vi "BMU参数读取-Auto.vi"(7 "Socket":dbl, 8 "CAN端口":u16(ring), 9 "设备索引号":u16(ring), 10 "CAN卡类型":u32(ring)=21, 11 "从板号":u8=1) -> (3 "成功?":bool)   [LabVIEW 2013] (continued)
                                tunnel: w3912 -> [w3927] mode=indexing
                                tunnel: [w3923] -> w3910 mode=indexing
                                n2326 = Equal To 0?(x=w3927) -> (x = 0?=w3926:bool)
                                n2327 = Select(t="无", s=w3926, f="故障") -> (s? t:f=w3923:string)
                                }
                                n2328 = Insert Into Array(array=w3911, new element=w3910) -> (w3909:string[])  [unwired: 1 in]
                              }
                              n2329 = call "详细故障分解.vi"("名称"=string[] ["初始化失败(RS232)", "发送异常(RS232)", "接收异常(RS232)", "总线超时(RS232)", "初始化失败(RS485)", "发送异常(RS485)", "接收异常(RS485)", "总线超时(RS485)"], "故障输入口"=w3903) -> ("输出数组"=w3901:string[][])  [unwired: 1 in, 2 out]
                              n2330 = local write "电池故障"(w3901) -> ()
                            }
                            frame 6 {
                              n2331 = for {
                                N: 2 -> [_]
                                tunnel: w3932 -> [w3949]
                                shift-right: [w3936] -> w3930
                                shift-left: string[] [] -> [w3938]
                                i -> [w3935]
                                w3943 = 8 ("索引")
                                w3947 = 2 ("y")
                                n2332 = Multiply(x=w3935, y=w3947) -> (x*y=w3948:i32)
                                n2333 = Array Subset(array=w3949, index=w3948, length=w3947) -> (w3946:u8[])
                                n2334 = Index Array(array=w3946) -> (element #1=w3945:u8, element #2=w3944:u8)  [unwired: 2 in]
                                n2335 = call "二进制解析-8.6.vi"("索引"=w3943, "数值"=w3945) -> ("低位子数组"=w3942:i32[])  [unwired: 1 in, 2 out]
                                n2336 = call "二进制解析-8.6.vi"("索引"=w3943, "数值"=w3944) -> ("低位子数组"=w3941:i32[])  [unwired: 1 in, 2 out]
                                n2337 = Insert Into Array(array=w3942, new element=w3941) -> (w3940:i32[])  [unwired: 1 in]
                                n2338 = Reverse 1D Array(array=w3940) -> (reversed array=w3939:i32[])
                                n2339 = for {
                                N: 16 -> [_]
                                tunnel: w3939 -> [w3954] mode=indexing
                                tunnel: [w3950] -> w3937 mode=indexing
                                n2340 = Equal To 0?(x=w3954) -> (x = 0?=w3953:bool)
                                n2341 = Select(t="无", s=w3953, f="故障") -> (s? t:f=w3950:string)
                                }
                                n2342 = Insert Into Array(array=w3938, new element=w3937) -> (w3936:string[])  [unwired: 1 in]
                              }
                              n2343 = call "详细故障分解.vi"("名称"=string[] ["DI1对地短", "DI1对电源短", "DI2对地短", "DI2对电源短", "DI3对地短", "DI3对电源短", "DI4对地短", "DI4对电源短", "DI5对地短", "DI5对电源短", "DI6对地短", "DI6对电源短", "DI7对地短", "DI7对电源短", "DI8对地短", "DI8对电源短", "DO1对地短", "DO1对电源短", "DO2对地短", "DO2对电源短", "DO3对地短", "DO3对电源短", "DO4对地短", "DO4对电源短", "DO5对地短", "DO5对电源短", "DO6对地短", "DO6对电源短", "DO7对地短", "DO7对电源短", "DO8对地短", "DO8对电源短"], "故障输入口"=w3930) -> ("输出数组"=w3928:string[][])  [unwired: 1 in, 2 out]
                              n2344 = local write "电池故障"(w3928) -> ()
                            }
                            frame 7 {
                              n2345 = for {
                                N: 2 -> [_]
                                tunnel: w3959 -> [w3976]
                                shift-right: [w3963] -> w3957
                                shift-left: string[] [] -> [w3965]
                                i -> [w3961]
                                w3970 = 8 ("索引")
                                w3974 = 2 ("y")
                                n2346 = Multiply(x=w3961, y=w3974) -> (x*y=w3975:i32)
                                n2347 = Array Subset(array=w3976, index=w3975, length=w3974) -> (w3973:u8[])
                                n2348 = Index Array(array=w3973) -> (element #1=w3972:u8, element #2=w3971:u8)  [unwired: 2 in]
                                n2349 = call "二进制解析-8.6.vi"("索引"=w3970, "数值"=w3972) -> ("低位子数组"=w3969:i32[])  [unwired: 1 in, 2 out]
                                n2350 = call "二进制解析-8.6.vi"("索引"=w3970, "数值"=w3971) -> ("低位子数组"=w3968:i32[])  [unwired: 1 in, 2 out]
                                n2351 = Insert Into Array(array=w3969, new element=w3968) -> (w3967:i32[])  [unwired: 1 in]
                                n2352 = case shown="1" w3961 {
                                tunnel: [4 6] -> w3962
                                frame 0, Default {
                                }
                                frame 1 {
                                }
                                }
                                n2353 = Reverse 1D Array(array=w3967) -> (reversed array=w3966:i32[])
                                n2354 = for {
                                N: w3962 -> [_]
                                tunnel: w3966 -> [w3983] mode=indexing
                                tunnel: [w3979] -> w3964 mode=indexing
                                n2355 = Equal To 0?(x=w3983) -> (x = 0?=w3982:bool)
                                n2356 = Select(t="无", s=w3982, f="故障") -> (s? t:f=w3979:string)
                                }
                                n2357 = Insert Into Array(array=w3965, new element=w3964) -> (w3963:string[])  [unwired: 1 in]
                              }
                              n2358 = call "详细故障分解.vi"("名称"=string[] ["超时(pre-chg)", "后端开路(pre-chg)", "后端短路(pre-chg)", "预充电回路断开(pre-chg)", "正级继电器驱动故障(relay_driver)", "负级继电器驱动故障(relay_driver)", "预充电继电器驱动故障(relay_driver)", "充电继电器驱动故障(relay_driver)", "风机继电器驱动故障(relay_driver)", "加热继电器驱动故障(relay_driver)"], "故障输入口"=w3957) -> ("输出数组"=w3955:string[][])  [unwired: 1 in, 2 out]
                              n2359 = local write "电池故障"(w3955) -> ()
                            }
                          }
                        }
                        frame True {
                          n2360 = Index Array(array=w3987, index #1=0 ("索引"), index #2=1 ("索引")) -> (element #1=w3990:u8, element #2=w3991:u8)
                          n2361 = Join Numbers(hi=w3990, lo=w3991) -> ((hi.lo)=w3989:u16)
                          n2362 = Number To Hexadecimal String(2:w3989) -> (0:w3988:string)  [unwired: 1 out]
                          n2363 = Concatenate Strings("读取错误，代码： " ("字符串"), "0x" ("字符串"), w3988) -> (w3986:string)
                          n2364 = One Button Dialog(message=w3986, button name ("OK")="是" ("按钮名称（“确定”）")) -> ()  [unwired: 1 out]
                        }
                      }
                      n2365 = local write "消除"(FALSE ("消除")) -> ()
                      n2366 = global write "EV05全局变量1.vi" "流控帧 2"(FALSE ("流控帧 2")) -> ()
                      n2367 = local write "控制1"(FALSE ("控制1")) -> ()
                      n2368 = global write "EV05全局变量1.vi" "写入超时"(TRUE ("写入超时")) -> ()
                    }
                  }
                }
              }
            }
          }
        }
      }
      frame Error {
      }
    }
  }
  n2369 = disable-structure shown="启用" {
    disable-tunnel: w37 -> [w4002 _]
    disable-tunnel: w29 -> [w3997 _]
    disable-tunnel: w26 -> [w3996 _]
    disable-tunnel: w6 -> [w3995 _]
    frame Disabled {
      n2370 = while {
        tunnel: w4002 -> [w4011]
        tunnel: w3995 -> [w4010]
        tunnel: [w4009] -> w4001
        tunnel: [w4008] -> w4000
        tunnel: w3997 -> [_]
        tunnel: w3996 -> [_]
        stop <- w4007 stop-if-true
        n2371 = event shown="[49] \"全部读取\": 值改变" {
          selector: _ -> [_ _ _ _ _ _ _ _ _ _ _ _ _ _ _ _ _ _ _ _ _ _ _ _ _ _ _ _ _ _ _ _ _ _ _ _ _ _ _ _ _ _ _ _ _ _ _ _ _ _ _ _ _]
          dyn-events: _ -> [_ _ _ _ _ _ _ _ _ _ _ _ _ _ _ _ _ _ _ _ _ _ _ _ _ _ _ _ _ _ _ _ _ _ _ _ _ _ _ _ _ _ _ _ _ _ _ _ _ _ _ _ _]
          timeout: 200 -> [_ _ _ _ _ _ _ _ _ _ _ _ _ _ _ _ _ _ _ _ _ _ _ _ _ _ _ _ _ _ _ _ _ _ _ _ _ _ _ _ _ _ _ _ _ _ _ _ _ _ _ _ _]
          tunnel: [_ w4014 w4054 _ _ _ _ _ _ _ _ _ _ _ _ _ _ _ _ _ _ _ _ _ _ _ _ _ _ _ _ _ _ _ _ _ _ _ _ _ _ _ _ _ _ _ _ _ _ _ _ _ _] -> w4006
          tunnel: w4011 -> [w4013 w4017 w4053 _ w4094 w4105 w4116 w4127 w4132 w4143 w4154 w4165 w4176 w4187 w4204 w4215 w4231 w4769 w5191 w5216 w5244 w5347 w5420 w5432 w5442 w5488 _ _ w5538 w5605 w5672 w5739 w5806 w5873 w5940 w6008 w6076 w6143 w6210 w6280 w6291 w6330 w6352 w6392 w6414 w6452 w6512 w6547 w6583 w6616 w6685 w6718 w6751]
          tunnel: w4010 -> [w4012 w4016 w4052 _ w4093 w4104 w4115 w4126 w4131 w4142 w4153 w4164 w4175 w4186 w4203 w4214 w4230 w4768 w5190 w5215 w5243 w5346 w5418 w5430 w5441 w5487 _ _ w5537 w5604 w5671 w5738 w5805 w5872 w5939 w6007 w6075 w6142 w6209 w6278 w6290 w6329 w6351 w6391 w6413 w6451 w6511 w6546 w6582 w6615 w6684 w6717 w6750]
          tunnel: [w4013 w4017 w4053 _ w4094 w4105 w4116 w4127 w4132 w4143 w4154 w4165 w4176 w4187 w4204 w4215 w4231 w4769 w5191 w5216 w5244 w5347 w5419 w5431 w5442 w5488 _ _ w5538 w5605 w5672 w5739 w5806 w5873 w5940 w6008 w6076 w6143 w6210 w6279 w6289 w6328 w6350 w6390 w6412 w6452 w6510 w6545 w6581 w6614 w6683 w6716 w6749] -> w4009
          tunnel: [w4012 w4016 w4052 _ w4093 w4104 w4115 w4126 w4131 w4142 w4153 w4164 w4175 w4186 w4203 w4214 w4230 w4768 w5190 w5215 w5243 w5346 w5417 w5429 w5441 w5487 _ _ w5537 w5604 w5671 w5738 w5805 w5872 w5939 w6007 w6075 w6142 w6209 w6277 w6288 w6327 w6349 w6389 w6411 w6451 w6509 w6544 w6580 w6613 w6682 w6715 w6748] -> w4008
          tunnel: [_ _ _ _ _ _ _ _ _ _ _ _ _ _ _ _ _ _ _ _ _ _ _ _ _ _ _ _ _ _ _ _ _ _ _ _ _ _ _ _ w6288 w6327 w6349 w6389 w6411 _ w6509 w6544 w6580 w6613 w6682 w6715 w6748] -> w4005
          event Timeout {
            n2372 = event-data() -> ()  [unwired: 3 out]
          }
          event "停止": Value Change {
            n2373 = event-data() -> ("NewVal"=w4015:bool)  [unwired: 5 out]
            n2374 = stacked-sequence {
              tunnel: w4015 -> [w4034 _]
              tunnel: [w4034 _] -> w4014
              frame #0 {
                n2375 = global read "配置文件全局.vi" "诊断标定读取地址"() -> (w4018:path)
                n2376 = call <vilib>:"Application Directory.vi"() -> ("Application Directory"=w4028:path)
                n2377 = property class="VI"("FP.State"=T30."Hidden" ("前面板窗口:状态")) -> (reference out=w4030:refnum<vi>, error out=w4029:errorcluster)  [unwired: 2 in]
                n2378 = Build Path(base path=w4028, name or relative path="config.ini" ("名称或相对路径")) -> (appended path=w4026:path)
                n2379 = call <vilib>:"Open Config Data.vi"("configuration file path"=w4026) -> ("error out"=w4023:errorcluster, "refnum"=w4025:T26)  [unwired: 8 in, 1 out]
                n2380 = local write "停止"(TRUE ("停止")) -> ()
                n2381 = property class="VI"(reference=w4030, error in=w4029, "Front Panel.Open"=FALSE ("前面板窗口:打开")) -> ()  [unwired: 2 out]
                n2382 = call-poly <vilib>:"Write Key.vi"("section"="总信息", "error in (no error)"=w4023, "value"=w4018, "key"="诊断标定读取地址" ("section"), "refnum"=w4025) -> ("error out"=w4022:errorcluster, "refnum out"=w4021:T26)  [unwired: 4 in, 1 out]
                n2383 = call <vilib>:"Close Config Data.vi"("error in (no error)"=w4022, "refnum"=w4021) -> ("error out"=w4020:errorcluster)  [unwired: 8 in, 1 out]
                n2384 = call <vilib>:"Clear Errors.vi"("error in (no error)"=w4020) -> ()  [unwired: 6 in, 1 out]
              }
              frame #1 {
                n2385 = disable-structure shown="禁用" {
                  frame Disabled {
                    n2386 = local read "设备索引号"() -> (w4040:u16)
                    n2387 = local read "CAN卡类型"() -> (w4041:u32)
                    n2388 = local read "CAN端口"() -> (w4039:u16)
                    n2389 = Build Array(7) -> (w4036:i32[])
                    n2390 = call "transmit-8.6.vi"("can卡类型"=w4041, "设备索引号"=w4040, "CAN端口"=w4039, "ID"=418398080, "SendType"=u8 0, "Data"=w4036) -> ()  [unwired: 3 in, 11 out]
                  }
                  frame Enabled {
                    w4048 = u8 0 items=["Normal", "Listen Only"] ("工作方式")
                    w4047 = u8 1 items=["Dual Filter", "Single Filter"] ("滤波方式")
                    n2391 = local read "设备索引号"() -> (w4043:u16)
                    n2392 = local read "CAN卡类型"() -> (w4042:u32)
                    n2393 = local read "CAN端口"() -> (w4044:u16)
                    n2394 = call "CAN_Init-8.6.vi"("CAN卡类型"=w4042, "设备索引号"=w4043, "CAN端口"=w4044, "操作类型"=enum16{"初始化CAN", "关闭CAN"}."初始化CAN", "滤波方式"=w4047, "Accept Code"=u32 0, "簇"=T22 {"打开CAN"=FALSE, "初始化CAN"=TRUE, "开始CAN"=TRUE, "重启"=FALSE, "关闭CAN"=FALSE}, "Mask Code"=u32 4294967295 ("Accept Code"), "工作方式"=w4048, "是否滤波"=FALSE) -> ()  [unwired: 4 in, 6 out]
                  }
                }
              }
            }
          }
          event Panel Close? {
            n2395 = event-data() -> ()  [unwired: 5 out]
            n2396 = stacked-sequence {
              tunnel: [w4067 _] -> w4054
              frame #0 {
                w4067 = TRUE ("前面板窗口:打开")
                n2397 = global read "配置文件全局.vi" "诊断标定读取地址"() -> (w4056:path)
                n2398 = call <vilib>:"Application Directory.vi"() -> ("Application Directory"=w4066:path)
                n2399 = property class="VI"("FP.State"=T30."Hidden" ("前面板窗口:状态")) -> (reference out=w4069:refnum<vi>, error out=w4068:errorcluster)  [unwired: 2 in]
                n2400 = Build Path(base path=w4066, name or relative path="config.ini" ("名称或相对路径")) -> (appended path=w4064:path)
                n2401 = call <vilib>:"Open Config Data.vi"("configuration file path"=w4064) -> ("error out"=w4061:errorcluster, "refnum"=w4063:T26)  [unwired: 8 in, 1 out]
                n2402 = property class="VI"(reference=w4069, error in=w4068, "Front Panel.Open"=FALSE ("前面板窗口:打开")) -> ()  [unwired: 2 out]
                n2403 = call-poly <vilib>:"Write Key.vi"("section"="总信息", "error in (no error)"=w4061, "value"=w4056, "key"="诊断标定读取地址" ("section"), "refnum"=w4063) -> ("error out"=w4060:errorcluster, "refnum out"=w4059:T26)  [unwired: 4 in, 1 out]
                n2404 = call <vilib>:"Close Config Data.vi"("error in (no error)"=w4060, "refnum"=w4059) -> ("error out"=w4058:errorcluster)  [unwired: 8 in, 1 out]
                n2405 = call <vilib>:"Clear Errors.vi"("error in (no error)"=w4058) -> ()  [unwired: 6 in, 1 out]
                n2406 = local write "强制终止读写标记"(TRUE ("强制终止读写标记")) -> ()
                n2407 = local write "停止"(w4067) -> ()
              }
              frame #1 {
                w4075 = u8 0 items=["Normal", "Listen Only"] ("工作方式")
                w4076 = u8 1 items=["Dual Filter", "Single Filter"] ("滤波方式")
                n2408 = local read "设备索引号"() -> (w4080:u16)
                n2409 = local read "CAN卡类型"() -> (w4081:u32)
                n2410 = local read "CAN端口"() -> (w4079:u16)
                n2411 = call "CAN_Init-8.6.vi"("CAN卡类型"=w4081, "设备索引号"=w4080, "CAN端口"=w4079, "操作类型"=enum16{"初始化CAN", "关闭CAN"}."初始化CAN", "滤波方式"=w4076, "Accept Code"=u32 0, "簇"=T22 {"打开CAN"=FALSE, "初始化CAN"=TRUE, "开始CAN"=TRUE, "重启"=FALSE, "关闭CAN"=FALSE}, "Mask Code"=u32 4294967295 ("Accept Code"), "工作方式"=w4075, "是否滤波"=FALSE) -> ()  [unwired: 4 in, 6 out]
              }
            }
            n2412 = event-data("Discard?"=w4054) -> ()  [unwired: 1 in, 1 out]
          }
          event "终止读写按钮": Value Change {
            n2413 = event-data() -> ("NewVal"=w4082:bool)  [unwired: 6 out]
            n2414 = case shown="真" w4082 {
              frame False {
              }
              frame True {
                n2415 = local write "强制终止读写标记"(TRUE ("强制终止读写标记")) -> ()
              }
            }
          }
          event "1": Value Change {
            w4091 = FALSE ("1")
            n2416 = event-data() -> ()  [unwired: 7 out]
            n2417 = local write "主板2"(T9."项目信息" ("主从板")) -> ()
            n2418 = Not(x=w4091) -> (.not. x?=w4090:bool)
            n2419 = local write "1"(w4090) -> ()
            n2420 = local write "1 2"(w4091) -> ()
            n2421 = local write "1 3"(w4091) -> ()
            n2422 = local write "1 4"(w4091) -> ()
            n2423 = local write "1 5"(w4091) -> ()
            n2424 = local write "1 11"(w4091) -> ()
            n2425 = global read "功能码全局.vi" "主板监控2"() -> (w4089:bool[])
            n2426 = Index Array(array=w4089, index=6 ("索引")) -> (element=w4084:bool)
            n2427 = Select(t=0, s=w4084, f=1) -> (s? t:f=w4085:i32)
            n2428 = property on="项目信息" class="Tbl (严格)"("Disabled"=w4085) -> ()  [unwired: 2 in, 2 out]
            n2429 = property on="电池实际容量(A)" class="DigNum (严格)"("Disabled"=w4085) -> ()  [unwired: 2 in, 2 out]
            n2430 = property on="使用者" class="DigNum (严格)"("Disabled"=w4085) -> ()  [unwired: 2 in, 2 out]
            n2431 = property on="SOH(%)" class="DigNum (严格)"("Disabled"=w4085) -> ()  [unwired: 2 in, 2 out]
            n2432 = property on="电池额定容量(A)" class="DigNum (严格)"("Disabled"=w4085) -> ()  [unwired: 2 in, 2 out]
            n2433 = property on="SOC(%)" class="DigNum (严格)"("Disabled"=w4085) -> ()  [unwired: 2 in, 2 out]
            n2434 = property on="项目信息2" class="Clust (严格)"("DisabledEnum"=w4085) -> ()  [unwired: 2 in, 2 out]
            n2435 = property on="系统时钟" class="Str"("Disabled"=w4085) -> ()  [unwired: 2 in, 2 out]
            n2436 = property on="配置文件版本" class="Str"("Disabled"=w4085) -> ()  [unwired: 2 in, 2 out]
            n2437 = property on="车架(牌)号" class="Str"("Disabled"=w4085) -> ()  [unwired: 2 in, 2 out]
            n2438 = property on="产品编号" class="Str"("Disabled"=w4085) -> ()  [unwired: 2 in, 2 out]
          }
          event "1 2": Value Change {
            w4102 = FALSE ("1")
            n2439 = event-data() -> ()  [unwired: 7 out]
            n2440 = local write "主板2"(T9."一级故障阀值" ("主从板")) -> ()
            n2441 = Not(x=w4102) -> (.not. x?=w4101:bool)
            n2442 = local write "1"(w4102) -> ()
            n2443 = local write "1 2"(w4101) -> ()
            n2444 = local write "1 3"(w4102) -> ()
            n2445 = local write "1 4"(w4102) -> ()
            n2446 = local write "1 5"(w4102) -> ()
            n2447 = local write "1 11"(w4102) -> ()
            n2448 = global read "功能码全局.vi" "主板监控2"() -> (w4100:bool[])
            n2449 = Index Array(array=w4100, index=6 ("索引")) -> (element=w4095:bool)
            n2450 = Select(t=0, s=w4095, f=1) -> (s? t:f=w4098:i32)
            n2451 = property on="一级故障" class="Clust (严格)"("DisabledEnum"=w4098) -> ()  [unwired: 2 in, 2 out]
          }
          event "1 3": Value Change {
            w4113 = FALSE ("1")
            n2452 = event-data() -> ()  [unwired: 7 out]
            n2453 = local write "主板2"(T9."二级故障阀值" ("主从板")) -> ()
            n2454 = Not(x=w4113) -> (.not. x?=w4112:bool)
            n2455 = local write "1"(w4113) -> ()
            n2456 = local write "1 2"(w4113) -> ()
            n2457 = local write "1 3"(w4112) -> ()
            n2458 = local write "1 4"(w4113) -> ()
            n2459 = local write "1 5"(w4113) -> ()
            n2460 = local write "1 11"(w4113) -> ()
            n2461 = global read "功能码全局.vi" "主板监控2"() -> (w4111:bool[])
            n2462 = Index Array(array=w4111, index=6 ("索引")) -> (element=w4107:bool)
            n2463 = Select(t=0, s=w4107, f=1) -> (s? t:f=w4106:i32)
            n2464 = property on="一级故障 2" class="Clust (严格)"("DisabledEnum"=w4106) -> ()  [unwired: 2 in, 2 out]
          }
          event "1 4": Value Change {
            w4124 = FALSE ("1")
            n2465 = event-data() -> ()  [unwired: 7 out]
            n2466 = local write "主板2"(T9."三级故障阀值" ("主从板")) -> ()
            n2467 = Not(x=w4124) -> (.not. x?=w4123:bool)
            n2468 = local write "1"(w4124) -> ()
            n2469 = local write "1 2"(w4124) -> ()
            n2470 = local write "1 3"(w4124) -> ()
            n2471 = local write "1 4"(w4123) -> ()
            n2472 = local write "1 5"(w4124) -> ()
            n2473 = local write "1 11"(w4124) -> ()
            n2474 = global read "功能码全局.vi" "主板监控2"() -> (w4122:bool[])
            n2475 = Index Array(array=w4122, index=6 ("索引")) -> (element=w4117:bool)
            n2476 = Select(t=0, s=w4117, f=1) -> (s? t:f=w4120:i32)
            n2477 = property on="一级故障 3" class="Clust (严格)"("DisabledEnum"=w4120) -> ()  [unwired: 2 in, 2 out]
          }
          event "1 5": Value Change {
            w4129 = FALSE ("1")
            n2478 = event-data() -> ()  [unwired: 7 out]
            n2479 = local write "主板2"(T9."控制参数" ("主从板")) -> ()
            n2480 = Not(x=w4129) -> (.not. x?=w4128:bool)
            n2481 = local write "1"(w4129) -> ()
            n2482 = local write "1 2"(w4129) -> ()
            n2483 = local write "1 3"(w4129) -> ()
            n2484 = local write "1 4"(w4129) -> ()
            n2485 = local write "1 5"(w4128) -> ()
            n2486 = local write "1 11"(w4129) -> ()
            n2487 = disable-structure shown="禁用" {
              frame Disabled {
                n2488 = global read "功能码全局.vi" "主板监控2"() -> (w4136:bool[])
                n2489 = Index Array(array=w4136, index=6 ("索引")) -> (element=w4134:bool)
                n2490 = Select(t=0, s=w4134, f=1) -> (s? t:f=w4133:i32)
                n2491 = property on="风机开启温度" class="DigNum (严格)"("Disabled"=w4133) -> ()  [unwired: 2 in, 2 out]
                n2492 = property on="风机关闭温度" class="DigNum (严格)"("Disabled"=w4133) -> ()  [unwired: 2 in, 2 out]
                n2493 = property on="加热开启温度" class="DigNum (严格)"("Disabled"=w4133) -> ()  [unwired: 2 in, 2 out]
                n2494 = property on="加热关闭温度" class="DigNum (严格)"("Disabled"=w4133) -> ()  [unwired: 2 in, 2 out]
                n2495 = property on="风机开启温差" class="DigNum (严格)"("Disabled"=w4133) -> ()  [unwired: 2 in, 2 out]
                n2496 = property on="风机关闭温差" class="DigNum (严格)"("Disabled"=w4133) -> ()  [unwired: 2 in, 2 out]
                n2497 = property on="加热控制参数" class="Clust (严格)"("DisabledEnum"=w4133) -> ()  [unwired: 2 in, 2 out]
                n2498 = property on="最大允许总电压" class="DigNum (严格)"("Disabled"=w4133) -> ()  [unwired: 2 in, 2 out]
                n2499 = property on="最大允许充电温度" class="DigNum (严格)"("Disabled"=w4133) -> ()  [unwired: 2 in, 2 out]
                n2500 = property on="最小允许充电温度" class="DigNum (严格)"("Disabled"=w4133) -> ()  [unwired: 2 in, 2 out]
                n2501 = property on="电流步长" class="DigNum (严格)"("Disabled"=w4133) -> ()  [unwired: 2 in, 2 out]
                n2502 = property on="最大允许单体电压" class="DigNum (严格)"("Disabled"=w4133) -> ()  [unwired: 2 in, 2 out]
                n2503 = property on="最小允许单体电压" class="DigNum (严格)"("Disabled"=w4133) -> ()  [unwired: 2 in, 2 out]
                n2504 = property on="最大允许充电电流" class="DigNum (严格)"("Disabled"=w4133) -> ()  [unwired: 2 in, 2 out]
                n2505 = property on="最小允许充电电流" class="DigNum (严格)"("Disabled"=w4133) -> ()  [unwired: 2 in, 2 out]
              }
              frame Enabled {
              }
            }
          }
          event "1 11": Value Change {
            w4140 = FALSE ("1")
            n2506 = event-data() -> ()  [unwired: 7 out]
            n2507 = local write "主板2"(T9."电池信息" ("主从板")) -> ()
            n2508 = Not(x=w4140) -> (.not. x?=w4139:bool)
            n2509 = local write "1"(w4140) -> ()
            n2510 = local write "1 2"(w4140) -> ()
            n2511 = local write "1 3"(w4140) -> ()
            n2512 = local write "1 4"(w4140) -> ()
            n2513 = local write "1 5"(w4140) -> ()
            n2514 = local write "1 11"(w4139) -> ()
            n2515 = disable-structure shown="禁用" {
              frame Disabled {
                n2516 = global read "功能码全局.vi" "主板监控2"() -> (w4146:bool[])
                n2517 = Index Array(array=w4146, index=6 ("索引")) -> (element=w4144:bool)
                n2518 = Select(t=0, s=w4144, f=1) -> (s? t:f=w4147:i32)
                n2519 = property on="电池串联" class="DigNum (严格)"("Disabled"=w4147) -> ()  [unwired: 2 in, 2 out]
                n2520 = property on="电池并联" class="DigNum (严格)"("Disabled"=w4147) -> ()  [unwired: 2 in, 2 out]
                n2521 = property on="电池包额定容量" class="DigNum (严格)"("Disabled"=w4147) -> ()  [unwired: 2 in, 2 out]
                n2522 = property on="电池包额定能量(kWh)" class="DigNum (严格)"("Disabled"=w4147) -> ()  [unwired: 2 in, 2 out]
                n2523 = property on="电池包额定总电压" class="DigNum (严格)"("Disabled"=w4147) -> ()  [unwired: 2 in, 2 out]
                n2524 = property on="实际容量" class="DigNum (严格)"("Disabled"=w4147) -> ()  [unwired: 2 in, 2 out]
                n2525 = property on="电池包组号" class="Str"("Disabled"=w4147) -> ()  [unwired: 2 in, 2 out]
                n2526 = property on="电池生产日期" class="Str"("Disabled"=w4147) -> ()  [unwired: 2 in, 2 out]
                n2527 = property on="电池厂家" class="Str"("Disabled"=w4147) -> ()  [unwired: 2 in, 2 out]
                n2528 = property on="电池类型" class="Str"("Disabled"=w4147) -> ()  [unwired: 2 in, 2 out]
                n2529 = property on="累计充电总安时" class="DigNum (严格)"("Disabled"=w4147) -> ()  [unwired: 2 in, 2 out]
                n2530 = property on="累计放电总安时" class="DigNum (严格)"("Disabled"=w4147) -> ()  [unwired: 2 in, 2 out]
                n2531 = property on="电池放空次数" class="DigNum (严格)"("Disabled"=w4147) -> ()  [unwired: 2 in, 2 out]
                n2532 = property on="电池充满次数" class="DigNum (严格)"("Disabled"=w4147) -> ()  [unwired: 2 in, 2 out]
                n2533 = property on="电池充电次数" class="DigNum (严格)"("Disabled"=w4147) -> ()  [unwired: 2 in, 2 out]
                n2534 = property on="电池信息" class="Clust (严格)"("DisabledEnum"=w4147) -> ()  [unwired: 2 in, 2 out]
              }
              frame Enabled {
              }
            }
          }
          event "1 6": Value Change {
            w4151 = FALSE ("1 6")
            n2535 = event-data() -> ()  [unwired: 7 out]
            n2536 = Not(x=w4151) -> (.not. x?=w4150:bool)
            n2537 = local write "1 6"(w4150) -> ()
            n2538 = local write "1 7"(w4151) -> ()
            n2539 = local write "1 8"(w4151) -> ()
            n2540 = local write "1 9"(w4151) -> ()
            n2541 = local write "1 10"(w4151) -> ()
            n2542 = local write "等级 2"(T20."从板信息" ("等级 2")) -> ()
            n2543 = disable-structure shown="禁用" {
              frame Disabled {
                n2544 = global read "功能码全局.vi" "主板监控2"() -> (w4157:bool[])
                n2545 = Index Array(array=w4157, index=6 ("索引")) -> (element=w4155:bool)
                n2546 = Select(t=0, s=w4155, f=1) -> (s? t:f=w4158:i32)
                n2547 = property on="项目信息 2" class="Tbl (严格)"("Disabled"=w4158) -> ()  [unwired: 2 in, 2 out]
                n2548 = property on="加热控制参数" class="Clust (严格)"("Disabled"=w4158) -> ()  [unwired: 2 in, 2 out]
              }
              frame Enabled {
              }
            }
          }
          event "1 7": Value Change {
            w4162 = FALSE ("1 6")
            n2549 = event-data() -> ()  [unwired: 7 out]
            n2550 = disable-structure shown="禁用" {
              frame Disabled {
                n2551 = global read "功能码全局.vi" "主板监控2"() -> (w4171:bool[])
                n2552 = Index Array(array=w4171, index=6 ("索引")) -> (element=w4166:bool)
                n2553 = Select(t=0, s=w4166, f=1) -> (s? t:f=w4167:i32)
                n2554 = property on="一级故障 6" class="Clust (严格)"("DisabledEnum"=w4167) -> ()  [unwired: 2 in, 2 out]
              }
              frame Enabled {
              }
            }
            n2555 = local write "等级 2"(T20."一级故障阀值" ("等级 2")) -> ()
            n2556 = Not(x=w4162) -> (.not. x?=w4161:bool)
            n2557 = local write "1 6"(w4162) -> ()
            n2558 = local write "1 7"(w4161) -> ()
            n2559 = local write "1 8"(w4162) -> ()
            n2560 = local write "1 9"(w4162) -> ()
            n2561 = local write "1 10"(w4162) -> ()
          }
          event "1 8": Value Change {
            w4173 = FALSE ("1 6")
            n2562 = event-data() -> ()  [unwired: 7 out]
            n2563 = disable-structure shown="禁用" {
              frame Disabled {
                n2564 = global read "功能码全局.vi" "主板监控2"() -> (w4182:bool[])
                n2565 = Index Array(array=w4182, index=6 ("索引")) -> (element=w4177:bool)
                n2566 = Select(t=0, s=w4177, f=1) -> (s? t:f=w4178:i32)
                n2567 = property on="一级故障 7" class="Clust (严格)"("DisabledEnum"=w4178) -> ()  [unwired: 2 in, 2 out]
              }
              frame Enabled {
              }
            }
            n2568 = local write "等级 2"(T20."二级故障阀值" ("等级 2")) -> ()
            n2569 = Not(x=w4173) -> (.not. x?=w4172:bool)
            n2570 = local write "1 6"(w4173) -> ()
            n2571 = local write "1 7"(w4173) -> ()
            n2572 = local write "1 8"(w4172) -> ()
            n2573 = local write "1 9"(w4173) -> ()
            n2574 = local write "1 10"(w4173) -> ()
          }
          event "1 9": Value Change {
            w4184 = FALSE ("1 6")
            n2575 = event-data() -> ()  [unwired: 7 out]
            n2576 = disable-structure shown="禁用" {
              frame Disabled {
                n2577 = global read "功能码全局.vi" "主板监控2"() -> (w4193:bool[])
                n2578 = Index Array(array=w4193, index=6 ("索引")) -> (element=w4188:bool)
                n2579 = Select(t=0, s=w4188, f=1) -> (s? t:f=w4189:i32)
                n2580 = property on="一级故障 8" class="Clust (严格)"("DisabledEnum"=w4189) -> ()  [unwired: 2 in, 2 out]
              }
              frame Enabled {
              }
            }
            n2581 = local write "等级 2"(T20."三级故障阀值" ("等级 2")) -> ()
            n2582 = Not(x=w4184) -> (.not. x?=w4183:bool)
            n2583 = local write "1 6"(w4184) -> ()
            n2584 = local write "1 7"(w4184) -> ()
            n2585 = local write "1 8"(w4184) -> ()
            n2586 = local write "1 9"(w4183) -> ()
            n2587 = local write "1 10"(w4184) -> ()
          }
          event "1 10": Value Change {
            w4201 = FALSE ("1 6")
            n2588 = event-data() -> ()  [unwired: 7 out]
            n2589 = global read "功能码全局.vi" "主板监控2"() -> (w4199:bool[])
            n2590 = Index Array(array=w4199, index=6 ("索引")) -> (element=w4194:bool)
            n2591 = Select(t=0, s=w4194, f=1) -> (s? t:f=w4195:i32)
            n2592 = local write "等级 2"(T20."快换参数" ("等级 2")) -> ()
            n2593 = property on="电池组信息" class="Clust (严格)"("Disabled"=w4195) -> ()  [unwired: 2 in, 2 out]
            n2594 = Not(x=w4201) -> (.not. x?=w4200:bool)
            n2595 = local write "1 6"(w4201) -> ()
            n2596 = local write "1 7"(w4201) -> ()
            n2597 = local write "1 8"(w4201) -> ()
            n2598 = local write "1 9"(w4201) -> ()
            n2599 = local write "1 10"(w4200) -> ()
          }
          event "1 12": Value Change {
            w4206 = FALSE ("1 6")
            n2600 = event-data() -> ()  [unwired: 7 out]
            n2601 = global read "功能码全局.vi" "主板监控2"() -> (w4213:bool[])
            n2602 = Index Array(array=w4213, index=6 ("索引")) -> (element=w4209:bool)
            n2603 = Select(t=0, s=w4209, f=1) -> (s? t:f=w4205:i32)
            n2604 = local write "等级 2"(T15."均衡参数" ("等级 2")) -> ()
            n2605 = property on="均衡参数" class="Clust (严格)"("DisabledEnum"=w4205) -> ()  [unwired: 2 in, 2 out]
            n2606 = Not(x=w4206) -> (.not. x?=w4207:bool)
            n2607 = local write "1 12"(w4207) -> ()
            n2608 = local write "1 6"(w4206) -> ()
            n2609 = local write "1 7"(w4206) -> ()
            n2610 = local write "1 8"(w4206) -> ()
            n2611 = local write "1 9"(w4206) -> ()
            n2612 = local write "1 10"(w4206) -> ()
          }
          event "主板选项": Mouse Down {
            n2613 = event-data() -> ("CtlRef"=w4229:refnum<vi>)  [unwired: 8 out]
            n2614 = global read "功能码全局.vi" "主板监控2"() -> (w4218:bool[])
            n2615 = property class="Tree (严格)"(reference=w4229) -> ("Value"=w4221:string)  [unwired: 1 in, 2 out]
            n2616 = Index Array(array=w4218, index=6 ("索引")) -> (element=w4216:bool)
            n2617 = case shown="\"二维码\"" w4221 {
              tunnel: [T9."项目信息" ("主从板") T9."项目信息" ("主从板") T9."项目信息" ("主从板") T9."项目信息" ("主从板") T9."项目信息" ("主从板") T9."项目信息" ("主从板") T9."项目信息" ("主从板") T9."项目信息" ("主从板") T9."项目信息" ("主从板") T9."项目信息" ("主从板") T9."项目信息" ("主从板") T9."项目信息" ("主从板") T9."项目信息" ("主从板") T9."项目信息" ("主从板") T9."项目信息" ("主从板") T9."项目信息" ("主从板") T9."二级故障阀值" ("主从板") T9."三级故障阀值" ("主从板") T9."一级故障阀值" ("主从板") T9."控制参数" ("主从板") T9."控制参数" ("主从板") T9."电池信息" ("主从板") T9."电池信息" ("主从板") T9."电池信息" ("主从板") T9."电池信息" ("主从板") T9."电池信息" ("主从板") T9."项目信息" ("主从板")] -> w4228
              tunnel: [w4239 w4246 w4261 w4276 w4293 w4333 w4367 w4414 w4452 w4502 w4537 w4551 w4566 w4581 w4596 w4610 w4623 w4637 w4650 w4664 w4678 w4691 w4705 w4719 w4733 w4747 w4751] -> w4227
              tunnel: [w4240 w4247 w4262 w4277 w4294 w4334 w4368 w4415 w4453 w4503 w4538 w4552 w4567 w4582 w4597 w4611 w4623 w4637 w4649 w4664 w4678 w4691 w4705 w4719 w4733 w4747 w4752] -> w4226
              tunnel: [w4240 w4247 w4262 w4277 w4294 w4334 w4368 w4415 w4453 w4503 w4538 w4552 w4567 w4582 w4597 w4611 w4624 w4637 w4650 w4664 w4678 w4691 w4705 w4719 w4733 w4747 w4752] -> w4225
              tunnel: [w4240 w4247 w4262 w4277 w4294 w4334 w4368 w4415 w4453 w4503 w4538 w4552 w4567 w4582 w4597 w4611 w4623 w4636 w4650 w4664 w4678 w4691 w4705 w4719 w4733 w4747 w4752] -> w4224
              tunnel: [w4240 w4247 w4262 w4277 w4294 w4334 w4368 w4415 w4453 w4503 w4538 w4552 w4567 w4582 w4597 w4611 w4623 w4637 w4650 w4663 w4677 w4691 w4705 w4719 w4733 w4747 w4752] -> w4223
              tunnel: [w4240 w4247 w4262 w4277 w4294 w4334 w4368 w4415 w4453 w4503 w4538 w4552 w4567 w4582 w4597 w4611 w4623 w4637 w4650 w4664 w4678 w4690 w4704 w4718 w4732 w4746 w4752] -> w4222
              tunnel: [w4232 FALSE w4257 w4272 w4285 w4325 w4358 w4405 w4444 w4495 w4532 w4546 w4560 w4574 w4589 w4605 w4619 w4632 w4645 w4659 w4672 w4686 w4699 w4713 w4727 w4741 FALSE] -> w4220
              tunnel: [w4232 TRUE w4254 w4269 w4284 w4324 w4359 w4406 w4443 w4494 w4531 w4545 w4559 w4575 w4590 w4604 w4618 w4631 w4644 w4658 w4671 w4685 w4698 w4712 w4726 w4740 FALSE] -> w4219
              tunnel: w4216 -> [w4237 _ w4251 w4266 w4281 w4320 w4355 w4402 w4440 w4492 w4528 w4542 w4556 w4571 w4586 w4601 w4615 w4628 w4641 w4655 w4668 w4682 w4695 w4709 w4723 w4737 _]
              frame "项目信息" {
                w4240 = FALSE
                n2618 = Select(t=0, s=w4237, f=1) -> (s? t:f=w4235:i32)
                n2619 = property on="项目信息" class="Tbl (严格)"("Disabled"=w4235) -> ()  [unwired: 2 in, 2 out]
                n2620 = property on="电池实际容量(A)" class="DigNum (严格)"("Disabled"=w4235) -> ()  [unwired: 2 in, 2 out]
                n2621 = property on="使用者" class="DigNum (严格)"("Disabled"=w4235) -> ()  [unwired: 2 in, 2 out]
                n2622 = property on="SOH(%)" class="DigNum (严格)"("Disabled"=w4235) -> ()  [unwired: 2 in, 2 out]
                n2623 = property on="从板个数" class="DigNum (严格)"("NumText.BGColor"=u32 6618880) -> ()  [unwired: 2 in, 2 out]
                n2624 = property on="电池额定容量(A)" class="DigNum (严格)"("Disabled"=w4235) -> ()  [unwired: 2 in, 2 out]
                n2625 = property on="SOC(%)" class="DigNum (严格)"("Disabled"=w4235) -> ()  [unwired: 2 in, 2 out]
                n2626 = property on="项目信息2" class="Clust (严格)"("DisabledEnum"=w4235) -> ()  [unwired: 2 in, 2 out]
                n2627 = property on="系统时钟" class="Str"("Disabled"=w4235) -> ()  [unwired: 2 in, 2 out]
                n2628 = property on="配置文件版本" class="Str"("Disabled"=w4235) -> ()  [unwired: 2 in, 2 out]
                n2629 = property on="车架(牌)号" class="Str"("Disabled"=w4235) -> ()  [unwired: 2 in, 2 out]
                n2630 = property on="产品编号" class="Str"("Disabled"=w4235) -> ()  [unwired: 2 in, 2 out]
                n2631 = local read "项目信息结果"() -> (w4233:bool)
                n2632 = Not(x=w4233) -> (.not. x?=w4232:bool)
                n2633 = Not(x=w4240) -> (.not. x?=w4239:bool)
              }
              frame "校正时钟" {
                w4243 = 2
                w4247 = FALSE
                n2634 = property on="从板个数" class="DigNum (严格)"("NumText.BGColor"=u32 13816530) -> ()  [unwired: 2 in, 2 out]
                n2635 = property on="项目信息" class="Tbl (严格)"("Disabled"=w4243) -> ()  [unwired: 2 in, 2 out]
                n2636 = property on="电池实际容量(A)" class="DigNum (严格)"("Disabled"=w4243) -> ()  [unwired: 2 in, 2 out]
                n2637 = property on="使用者" class="DigNum (严格)"("Disabled"=w4243) -> ()  [unwired: 2 in, 2 out]
                n2638 = property on="SOH(%)" class="DigNum (严格)"("Disabled"=w4243) -> ()  [unwired: 2 in, 2 out]
                n2639 = property on="电池额定容量(A)" class="DigNum (严格)"("Disabled"=w4243) -> ()  [unwired: 2 in, 2 out]
                n2640 = property on="SOC(%)" class="DigNum (严格)"("Disabled"=w4243) -> ()  [unwired: 2 in, 2 out]
                n2641 = property on="系统时钟" class="Str"("Disabled"=w4243) -> ()  [unwired: 2 in, 2 out]
                n2642 = property on="配置文件版本" class="Str"("Disabled"=w4243) -> ()  [unwired: 2 in, 2 out]
                n2643 = property on="车架(牌)号" class="Str"("Disabled"=w4243) -> ()  [unwired: 2 in, 2 out]
                n2644 = property on="项目信息2" class="Clust (严格)"("DisabledEnum"=w4243) -> ()  [unwired: 2 in, 2 out]
                n2645 = property on="产品编号" class="Str"("Disabled"=w4243) -> ()  [unwired: 2 in, 2 out]
                n2646 = Not(x=w4247) -> (.not. x?=w4246:bool)
              }
              frame "产品编号" {
                w4260 = 2
                w4262 = FALSE
                n2647 = property on="项目信息" class="Tbl (严格)"("Disabled"=w4260) -> ()  [unwired: 2 in, 2 out]
                n2648 = property on="电池实际容量(A)" class="DigNum (严格)"("Disabled"=w4260) -> ()  [unwired: 2 in, 2 out]
                n2649 = property on="使用者" class="DigNum (严格)"("Disabled"=w4260) -> ()  [unwired: 2 in, 2 out]
                n2650 = Select(t=0, s=w4251, f=1) -> (s? t:f=w4250:i32)
                n2651 = property on="SOH(%)" class="DigNum (严格)"("Disabled"=w4260) -> ()  [unwired: 2 in, 2 out]
                n2652 = property on="电池额定容量(A)" class="DigNum (严格)"("Disabled"=w4260) -> ()  [unwired: 2 in, 2 out]
                n2653 = property on="SOC(%)" class="DigNum (严格)"("Disabled"=w4260) -> ()  [unwired: 2 in, 2 out]
                n2654 = property on="产品编号" class="Str"("Disabled"=w4250) -> ()  [unwired: 2 in, 2 out]
                n2655 = property on="项目信息2" class="Clust (严格)"("DisabledEnum"=w4250) -> ()  [unwired: 2 in, 2 out]
                n2656 = property on="系统时钟" class="Str"("Disabled"=w4260) -> ()  [unwired: 2 in, 2 out]
                n2657 = property on="配置文件版本" class="Str"("Disabled"=w4260) -> ()  [unwired: 2 in, 2 out]
                n2658 = property on="车架(牌)号" class="Str"("Disabled"=w4260) -> ()  [unwired: 2 in, 2 out]
                n2659 = property on="从板个数" class="DigNum (严格)"("NumText.BGColor"=u32 13816530) -> ()  [unwired: 2 in, 2 out]
                n2660 = global read "功能码全局.vi" "主板项目信息5"() -> (w4258:bool[])
                n2661 = global read "功能码全局.vi" "主板项目信息6"() -> (w4255:bool[])
                n2662 = Index Array(array=w4258, index=0 ("索引")) -> (element=w4257:bool)
                n2663 = Index Array(array=w4255, index=1 ("索引")) -> (element=w4254:bool)
                n2664 = Not(x=w4262) -> (.not. x?=w4261:bool)
              }
              frame "二维码" {
                w4275 = 2
                w4277 = FALSE
                n2665 = property on="项目信息" class="Tbl (严格)"("Disabled"=w4275) -> ()  [unwired: 2 in, 2 out]
                n2666 = property on="电池实际容量(A)" class="DigNum (严格)"("Disabled"=w4275) -> ()  [unwired: 2 in, 2 out]
                n2667 = property on="使用者" class="DigNum (严格)"("Disabled"=w4275) -> ()  [unwired: 2 in, 2 out]
                n2668 = Select(t=0, s=w4266, f=1) -> (s? t:f=w4265:i32)
                n2669 = property on="SOH(%)" class="DigNum (严格)"("Disabled"=w4275) -> ()  [unwired: 2 in, 2 out]
                n2670 = property on="电池额定容量(A)" class="DigNum (严格)"("Disabled"=w4275) -> ()  [unwired: 2 in, 2 out]
                n2671 = property on="SOC(%)" class="DigNum (严格)"("Disabled"=w4275) -> ()  [unwired: 2 in, 2 out]
                n2672 = property on="产品编号" class="Str"("Disabled"=w4265) -> ()  [unwired: 2 in, 2 out]
                n2673 = property on="项目信息2" class="Clust (严格)"("DisabledEnum"=w4265) -> ()  [unwired: 2 in, 2 out]
                n2674 = property on="系统时钟" class="Str"("Disabled"=w4275) -> ()  [unwired: 2 in, 2 out]
                n2675 = property on="配置文件版本" class="Str"("Disabled"=w4275) -> ()  [unwired: 2 in, 2 out]
                n2676 = property on="车架(牌)号" class="Str"("Disabled"=w4275) -> ()  [unwired: 2 in, 2 out]
                n2677 = property on="从板个数" class="DigNum (严格)"("NumText.BGColor"=u32 13816530) -> ()  [unwired: 2 in, 2 out]
                n2678 = global read "功能码全局.vi" "主板项目信息5"() -> (w4273:bool[])
                n2679 = global read "功能码全局.vi" "主板项目信息6"() -> (w4270:bool[])
                n2680 = Index Array(array=w4273, index=0 ("索引")) -> (element=w4272:bool)
                n2681 = Index Array(array=w4270, index=1 ("索引")) -> (element=w4269:bool)
                n2682 = Not(x=w4277) -> (.not. x?=w4276:bool)
              }
              frame "电压个数" {
                w4292 = 2
                w4294 = FALSE
                n2683 = local read "从板个数"() -> (w4291:dbl)
                n2684 = property on="从板个数" class="DigNum (严格)"("NumText.BGColor"=u32 6618880) -> ()  [unwired: 2 in, 2 out]
                n2685 = property on="电池实际容量(A)" class="DigNum (严格)"("Disabled"=w4292) -> ()  [unwired: 2 in, 2 out]
                n2686 = property on="使用者" class="DigNum (严格)"("Disabled"=w4292) -> ()  [unwired: 2 in, 2 out]
                n2687 = property on="SOH(%)" class="DigNum (严格)"("Disabled"=w4292) -> ()  [unwired: 2 in, 2 out]
                n2688 = property on="电池额定容量(A)" class="DigNum (严格)"("Disabled"=w4292) -> ()  [unwired: 2 in, 2 out]
                n2689 = property on="SOC(%)" class="DigNum (严格)"("Disabled"=w4292) -> ()  [unwired: 2 in, 2 out]
                n2690 = property on="系统时钟" class="Str"("Disabled"=w4292) -> ()  [unwired: 2 in, 2 out]
                n2691 = property on="配置文件版本" class="Str"("Disabled"=w4292) -> ()  [unwired: 2 in, 2 out]
                n2692 = property on="车架(牌)号" class="Str"("Disabled"=w4292) -> ()  [unwired: 2 in, 2 out]
                n2693 = property on="产品编号" class="Str"("Disabled"=w4292) -> ()  [unwired: 2 in, 2 out]
                n2694 = Select(t=0, s=w4281, f=1) -> (s? t:f=w4280:i32)
                n2695 = control-ref of="项目信息"() -> (w4290:refnum<vi>)
                n2696 = stacked-sequence {
                  tunnel: w4291 -> [_ w4301 w4311]
                  tunnel: w4290 -> [w4296 w4300 w4312]
                  frame #0 {
                    w4297 = 0
                    n2697 = Bundle(w4297, w4297) -> (w4299:cluster{i32, i32})  [unwired: 1 out]
                    n2698 = property class="Tbl (严格)"(reference=w4296, "Index Values"=w4299) -> (error out=w4298:errorcluster)  [unwired: 1 in, 1 out]
                    n2699 = call <vilib>:"Clear Errors.vi"("error in (no error)"=w4298) -> ()  [unwired: 7 out]
                  }
                  frame #1 {
                    n2700 = for {
                      N: 10 -> [_]
                      tunnel: w4300 -> [w4310]
                      tunnel: w4301 -> [w4305]
                      i -> [w4304]
                      n2701 = Compound Arithmetic op=ADD(0.0 ("值"), w4305, w4304) -> (w4307:dbl)
                      n2702 = Bundle(w4307, 0) -> (w4309:cluster{dbl, i32})  [unwired: 1 out]
                      n2703 = property class="Tbl (严格)"(reference=w4310, "Active Cell"=w4309, "Cell BG Color"=u32 16448250) -> ()  [unwired: 1 in, 2 out]
                    }
                  }
                  frame #2 {
                    n2704 = for {
                      N: w4311 -> [_]
                      tunnel: w4312 -> [w4313]
                      i -> [w4314]
                      n2705 = Bundle(w4314, 0) -> (w4318:cluster{i32, i32})  [unwired: 1 out]
                      n2706 = property class="Tbl (严格)"(reference=w4313, "Active Cell"=w4318, "Cell BG Color"=u32 6618880) -> (error out=w4315:errorcluster)  [unwired: 1 in, 1 out]
                      n2707 = call <vilib>:"Clear Errors.vi"("error in (no error)"=w4315) -> ()  [unwired: 7 out]
                    }
                  }
                }
                n2708 = property on="项目信息" class="Tbl (严格)"("Disabled"=w4280) -> ()  [unwired: 2 in, 2 out]
                n2709 = global read "功能码全局.vi" "主板项目信息5"() -> (w4288:bool[])
                n2710 = global read "功能码全局.vi" "主板项目信息6"() -> (w4286:bool[])
                n2711 = Index Array(array=w4288, index=1 ("索引")) -> (element=w4285:bool)
                n2712 = Index Array(array=w4286, index=2 ("索引")) -> (element=w4284:bool)
                n2713 = Not(x=w4294) -> (.not. x?=w4293:bool)
              }
              frame "通道电压数" {
                w4332 = 2
                w4334 = FALSE
                n2714 = property on="从板个数" class="DigNum (严格)"("NumText.BGColor"=u32 13816530) -> ()  [unwired: 2 in, 2 out]
                n2715 = property on="电池实际容量(A)" class="DigNum (严格)"("Disabled"=w4332) -> ()  [unwired: 2 in, 2 out]
                n2716 = property on="使用者" class="DigNum (严格)"("Disabled"=w4332) -> ()  [unwired: 2 in, 2 out]
                n2717 = property on="SOH(%)" class="DigNum (严格)"("Disabled"=w4332) -> ()  [unwired: 2 in, 2 out]
                n2718 = property on="电池额定容量(A)" class="DigNum (严格)"("Disabled"=w4332) -> ()  [unwired: 2 in, 2 out]
                n2719 = property on="SOC(%)" class="DigNum (严格)"("Disabled"=w4332) -> ()  [unwired: 2 in, 2 out]
                n2720 = local read "从板个数"() -> (w4330:dbl)
                n2721 = property on="系统时钟" class="Str"("Disabled"=w4332) -> ()  [unwired: 2 in, 2 out]
                n2722 = property on="配置文件版本" class="Str"("Disabled"=w4332) -> ()  [unwired: 2 in, 2 out]
                n2723 = property on="车架(牌)号" class="Str"("Disabled"=w4332) -> ()  [unwired: 2 in, 2 out]
                n2724 = property on="产品编号" class="Str"("Disabled"=w4332) -> ()  [unwired: 2 in, 2 out]
                n2725 = control-ref of="项目信息"() -> (w4331:refnum<vi>)
                n2726 = stacked-sequence {
                  tunnel: w4331 -> [w4341 w4344]
                  tunnel: w4330 -> [w4340 w4343]
                  frame #0 {
                    n2727 = Compound Arithmetic op=ADD(1.0 ("值"), w4340) -> (w4337:dbl)
                    n2728 = Bundle(w4337, 0) -> (w4339:cluster{dbl, i32})  [unwired: 1 out]
                    n2729 = property class="Tbl (严格)"(reference=w4341, "Index Values"=w4339) -> ()  [unwired: 1 in, 2 out]
                  }
                  frame #1 {
                    n2730 = for {
                      N: 20 -> [_]
                      tunnel: w4344 -> [w4352]
                      tunnel: w4343 -> [w4347]
                      i -> [w4346]
                      n2731 = Compound Arithmetic op=ADD(1.0 ("值"), w4347, w4346) -> (w4349:dbl)
                      n2732 = Bundle(w4349, 0) -> (w4351:cluster{dbl, i32})  [unwired: 1 out]
                      n2733 = property class="Tbl (严格)"(reference=w4352, "Active Cell"=w4351, "Cell BG Color"=u32 6618880) -> ()  [unwired: 1 in, 2 out]
                    }
                  }
                }
                n2734 = Select(t=0, s=w4320, f=1) -> (s? t:f=w4321:i32)
                n2735 = property on="项目信息" class="Tbl (严格)"("Disabled"=w4321) -> ()  [unwired: 2 in, 2 out]
                n2736 = global read "功能码全局.vi" "主板项目信息5"() -> (w4328:bool[])
                n2737 = global read "功能码全局.vi" "主板项目信息6"() -> (w4326:bool[])
                n2738 = Index Array(array=w4328, index=2 ("索引")) -> (element=w4325:bool)
                n2739 = Index Array(array=w4326, index=3 ("索引")) -> (element=w4324:bool)
                n2740 = Not(x=w4334) -> (.not. x?=w4333:bool)
              }
              frame "电压起始值" {
                w4366 = 2
                w4368 = FALSE
                n2741 = property on="从板个数" class="DigNum (严格)"("NumText.BGColor"=u32 13816530) -> ()  [unwired: 2 in, 2 out]
                n2742 = property on="电池实际容量(A)" class="DigNum (严格)"("Disabled"=w4366) -> ()  [unwired: 2 in, 2 out]
                n2743 = property on="使用者" class="DigNum (严格)"("Disabled"=w4366) -> ()  [unwired: 2 in, 2 out]
                n2744 = property on="SOH(%)" class="DigNum (严格)"("Disabled"=w4366) -> ()  [unwired: 2 in, 2 out]
                n2745 = property on="电池额定容量(A)" class="DigNum (严格)"("Disabled"=w4366) -> ()  [unwired: 2 in, 2 out]
                n2746 = property on="SOC(%)" class="DigNum (严格)"("Disabled"=w4366) -> ()  [unwired: 2 in, 2 out]
                n2747 = local read "从板个数"() -> (w4364:dbl)
                n2748 = property on="系统时钟" class="Str"("Disabled"=w4366) -> ()  [unwired: 2 in, 2 out]
                n2749 = property on="配置文件版本" class="Str"("Disabled"=w4366) -> ()  [unwired: 2 in, 2 out]
                n2750 = property on="车架(牌)号" class="Str"("Disabled"=w4366) -> ()  [unwired: 2 in, 2 out]
                n2751 = property on="产品编号" class="Str"("Disabled"=w4366) -> ()  [unwired: 2 in, 2 out]
                n2752 = control-ref of="项目信息"() -> (w4365:refnum<vi>)
                n2753 = stacked-sequence {
                  tunnel: w4365 -> [w4375 w4378 w4391]
                  tunnel: w4364 -> [w4374 w4377 w4390]
                  frame #0 {
                    n2754 = Compound Arithmetic op=ADD(21.0 ("值"), w4374) -> (w4371:dbl)
                    n2755 = Bundle(w4371, 0) -> (w4373:cluster{dbl, i32})  [unwired: 1 out]
                    n2756 = property class="Tbl (严格)"(reference=w4375, "Index Values"=w4373) -> ()  [unwired: 1 in, 2 out]
                  }
                  frame #1 {
                    n2757 = for {
                      N: 10 -> [_]
                      tunnel: w4378 -> [w4388]
                      tunnel: w4377 -> [w4383]
                      i -> [w4382]
                      n2758 = Multiply(x=w4383, y=2.0) -> (x*y=w4380:dbl)
                      n2759 = Compound Arithmetic op=ADD(21.0 ("值"), w4380, w4382) -> (w4385:dbl)
                      n2760 = Bundle(w4385, 0) -> (w4387:cluster{dbl, i32})  [unwired: 1 out]
                      n2761 = property class="Tbl (严格)"(reference=w4388, "Active Cell"=w4387, "Cell BG Color"=u32 16448250) -> ()  [unwired: 1 in, 2 out]
                    }
                  }
                  frame #2 {
                    n2762 = Increment(x=w4390) -> (x+1=w4389:dbl)
                    n2763 = for {
                      N: w4389 -> [_]
                      tunnel: w4391 -> [w4399]
                      tunnel: w4390 -> [w4394]
                      i -> [w4393]
                      n2764 = Compound Arithmetic op=ADD(21.0 ("值"), w4394, w4393) -> (w4396:dbl)
                      n2765 = Bundle(w4396, 0) -> (w4398:cluster{dbl, i32})  [unwired: 1 out]
                      n2766 = property class="Tbl (严格)"(reference=w4399, "Active Cell"=w4398, "Cell BG Color"=u32 6618880) -> ()  [unwired: 1 in, 2 out]
                    }
                  }
                }
                n2767 = Select(t=0, s=w4355, f=1) -> (s? t:f=w4354:i32)
                n2768 = property on="项目信息" class="Tbl (严格)"("Disabled"=w4354) -> ()  [unwired: 2 in, 2 out]
                n2769 = global read "功能码全局.vi" "主板项目信息5"() -> (w4362:bool[])
                n2770 = global read "功能码全局.vi" "主板项目信息6"() -> (w4360:bool[])
                n2771 = Index Array(array=w4362, index=3 ("索引")) -> (element=w4358:bool)
                n2772 = Index Array(array=w4360, index=4 ("索引")) -> (element=w4359:bool)
                n2773 = Not(x=w4368) -> (.not. x?=w4367:bool)
              }
              frame "温度个数" {
                w4413 = 2
                w4415 = FALSE
                n2774 = property on="电池实际容量(A)" class="DigNum (严格)"("Disabled"=w4413) -> ()  [unwired: 2 in, 2 out]
                n2775 = property on="使用者" class="DigNum (严格)"("Disabled"=w4413) -> ()  [unwired: 2 in, 2 out]
                n2776 = property on="SOH(%)" class="DigNum (严格)"("Disabled"=w4413) -> ()  [unwired: 2 in, 2 out]
                n2777 = property on="电池额定容量(A)" class="DigNum (严格)"("Disabled"=w4413) -> ()  [unwired: 2 in, 2 out]
                n2778 = property on="SOC(%)" class="DigNum (严格)"("Disabled"=w4413) -> ()  [unwired: 2 in, 2 out]
                n2779 = local read "从板个数"() -> (w4411:dbl)
                n2780 = control-ref of="项目信息"() -> (w4412:refnum<vi>)
                n2781 = stacked-sequence {
                  tunnel: w4412 -> [w4420 w4423 w4430]
                  tunnel: w4411 -> [w4417 w4422 w4429]
                  frame #0 {
                    n2782 = Bundle("从板个数"=w4417, 0) -> (w4419:cluster{"从板个数":dbl, i32})  [unwired: 1 out]
                    n2783 = property class="Tbl (严格)"(reference=w4420, "Index Values"=w4419) -> ()  [unwired: 1 in, 2 out]
                  }
                  frame #1 {
                    n2784 = for {
                      N: 20 -> [_]
                      tunnel: w4423 -> [w4428]
                      tunnel: w4422 -> [_]
                      i -> [w4424]
                      n2785 = Bundle(w4424, 0) -> (w4427:cluster{i32, i32})  [unwired: 1 out]
                      n2786 = property class="Tbl (严格)"(reference=w4428, "Active Cell"=w4427, "Cell BG Color"=u32 16448250) -> ()  [unwired: 1 in, 2 out]
                    }
                  }
                  frame #2 {
                    n2787 = for {
                      N: w4429 -> [_]
                      tunnel: w4430 -> [w4437]
                      tunnel: w4429 -> [w4431]
                      i -> [w4432]
                      n2788 = Compound Arithmetic op=ADD(w4431, w4432) -> (w4434:dbl)
                      n2789 = Bundle(w4434, 0) -> (w4436:cluster{dbl, i32})  [unwired: 1 out]
                      n2790 = property class="Tbl (严格)"(reference=w4437, "Active Cell"=w4436, "Cell BG Color"=u32 6618880) -> ()  [unwired: 1 in, 2 out]
                    }
                  }
                }
                n2791 = property on="系统时钟" class="Str"("Disabled"=w4413) -> ()  [unwired: 2 in, 2 out]
                n2792 = property on="配置文件版本" class="Str"("Disabled"=w4413) -> ()  [unwired: 2 in, 2 out]
                n2793 = property on="车架(牌)号" class="Str"("Disabled"=w4413) -> ()  [unwired: 2 in, 2 out]
                n2794 = property on="产品编号" class="Str"("Disabled"=w4413) -> ()  [unwired: 2 in, 2 out]
                n2795 = property on="从板个数" class="DigNum (严格)"("NumText.BGColor"=u32 13816530) -> ()  [unwired: 2 in, 2 out]
                n2796 = Select(t=0, s=w4402, f=1) -> (s? t:f=w4401:i32)
                n2797 = property on="项目信息" class="Tbl (严格)"("Disabled"=w4401) -> ()  [unwired: 2 in, 2 out]
